vi "Read Robot Speed Limit.vi"(8 "error in":errorcluster, 11 "Config Manager in":refnum<class "Config Manager Class.lvclass">) -> (0 "error out":errorcluster, 2 "Vec3d out":refnum<class "Vec3d Class.lvclass">, 3 "Config Manager out":refnum<class "Config Manager Class.lvclass">)   [LabVIEW 2011, in "Config Manager Class.lvclass"]
uses:
  Config Manager Class.lvclass
  Vec3d Class/Vec3d Class.lvclass
  Config Manager Class.lvclass/Config Manager Class.ctl
  <vilib>/Utility/config.llb/Read Key (String).vi
  <vilib>/Utility/config.llb/NI_LVConfig.lvlib
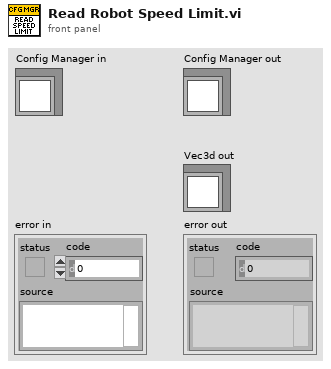
[diagram p1: front panel]
types:
  T1 = typedef "NI_LVConfig.lvlib/Config Data RefNum.ctl" = refnum<k1>
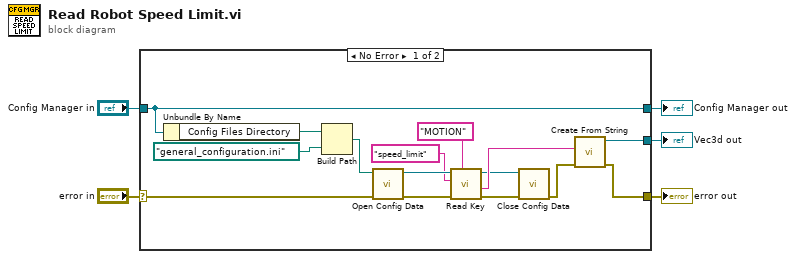
[diagram p0: block diagram]
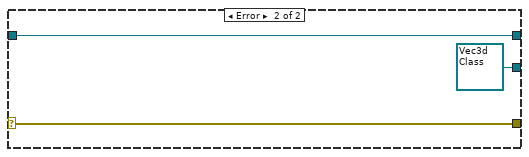
[diagram p2: hidden frame]
diagram:
  n1 = case shown="No Error" "error in" {
    selector: "error in" -> [w7 w23]
    tunnel: [w6 w23] -> w4
    tunnel: [w20 w22] -> w2
    tunnel: "Config Manager in" -> [w20 w22]
    tunnel: [w11 refnum<class "Vec3d Class.lvclass"> refnum ("Vec3d out")] -> w1
    frame No Error {
      n2 = Unbundle By Name(w20) -> ("Config Files Directory"=w19:path)
      n3 = Build Path(base path=w19, name or relative path=path "general_configuration.ini") -> (appended path=w17:path)
      n4 = call <vilib>:"Open Config Data.vi"("error in (no error)"=w7, "configuration file path"=w17) -> ("error out"=w15:errorcluster, "refnum"=w16:T1)  [unwired: 7 in, 1 out]
      n5 = call-poly <vilib>:"Read Key.vi"("section"="MOTION", "error in (no error)"=w15, "key"="speed_limit", "refnum"=w16) -> ("error out"=w9:errorcluster, "value"=w12:string, "refnum out"=w10:T1)  [unwired: 4 in, 1 out]
      n6 = call <vilib>:"Close Config Data.vi"("error in (no error)"=w9, "refnum"=w10) -> ("error out"=w8:errorcluster)  [unwired: 8 in, 1 out]
      n7 = call "Create From String.vi"("error in"=w8, "Input String"=w12) -> ("error out"=w6:errorcluster, "Vec3d out"=w11:refnum<class "Vec3d Class.lvclass">)  [unwired: 8 in]
    }
    frame Error {
    }
  }
  "error out" <- w4
  "Config Manager out" <- w2
  "Vec3d out" <- w1
